vi "synch tester RT.vi"() -> ()   [LabVIEW 2015]
uses:
  <vilib>/rvi/interface/nirviMethod/nirviMethod.xnode
  <vilib>/FPGAPlugInAG/Dynamic/niLvFpga_Run_Dynamic.vi
  <vilib>/FPGAPlugInAG/Dynamic/niLvFpga_ReadFifo_Dynamic.vi
  <vilib>/rvi/errors/niLvFpgaMergeErrorWithErrorCode.vi
  <vilib>/FPGAPlugInAG/Dynamic/niLvFpga_Abort_Dynamic.vi
  <vilib>/rvi/interface/nirviReadWriteControl/nirviReadWriteControl.xnode
  <vilib>/FPGAPlugInAG/Dynamic/niLvFpga_ConfigureFifo_Dynamic.vi
  <vilib>/rvi/interface/nirviOpenFPGA/nirviOpenFPGA.xnode
  <vilib>/FPGAPlugInAG/PXIe-7972R/niLvFpga_Open_PXIe-7972R.vi
  <vilib>/rvi/interface/common/dynamic/niFpgaDynamicAddResources.vi
  NiFpgaLv.dll
  <vilib>/Utility/error.llb/Error Cluster From Error Code.vi
  <vilib>/rvi/interface/Simulation/niFpgaSimulationCallBeginRW.vi
  <vilib>/rvi/errors/niLvFpgaAdjustHostInterfaceError.vi
  FPGA Bitfiles/GMLIDARV5.1_Master_TimingTestermast_BSVpvPZHDb8.lvbitx
  FPGA/Timing Tester master.vi
  FPGA Bitfiles/GMLIDARV5.1_Slave_TimingTesterslav_7ZC0ePWmfic.lvbitx
  FPGA/Timing Tester slave.vi
panel:
  in  "Number of Elements":u32
  out "Elements Remaining":u32
  out "error out 2":errorcluster
  out "error out":errorcluster
  in  "stop":bool
  out "Waveform Graph":i16[](graph)
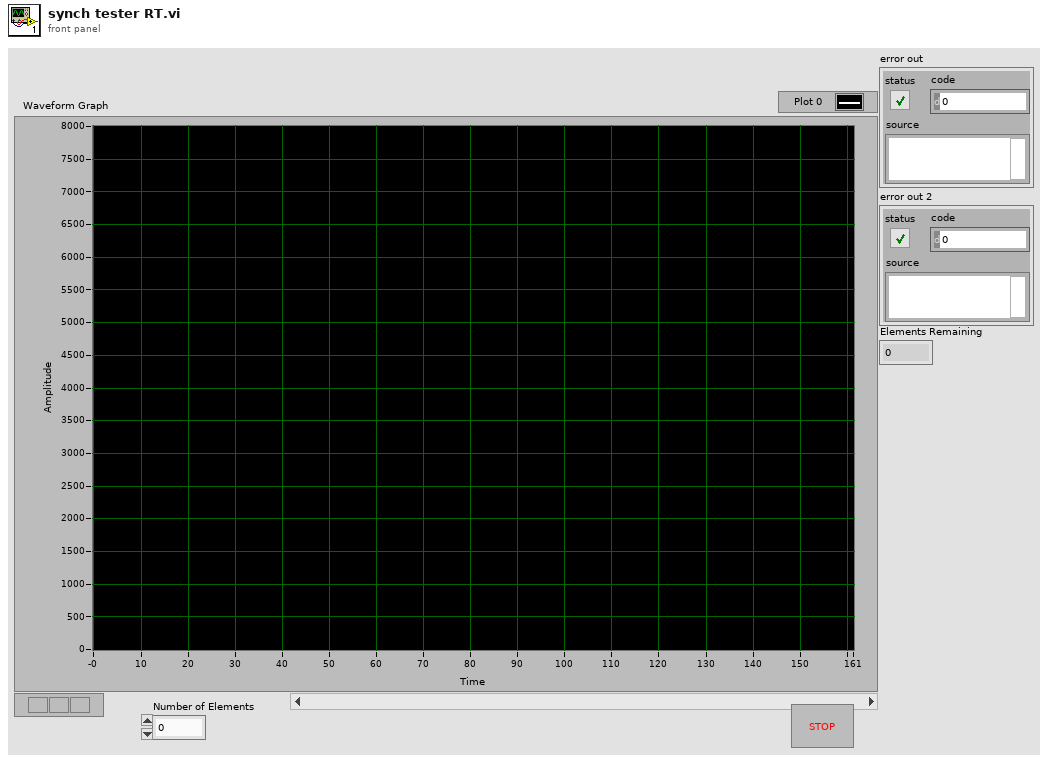
[diagram p1: front panel]
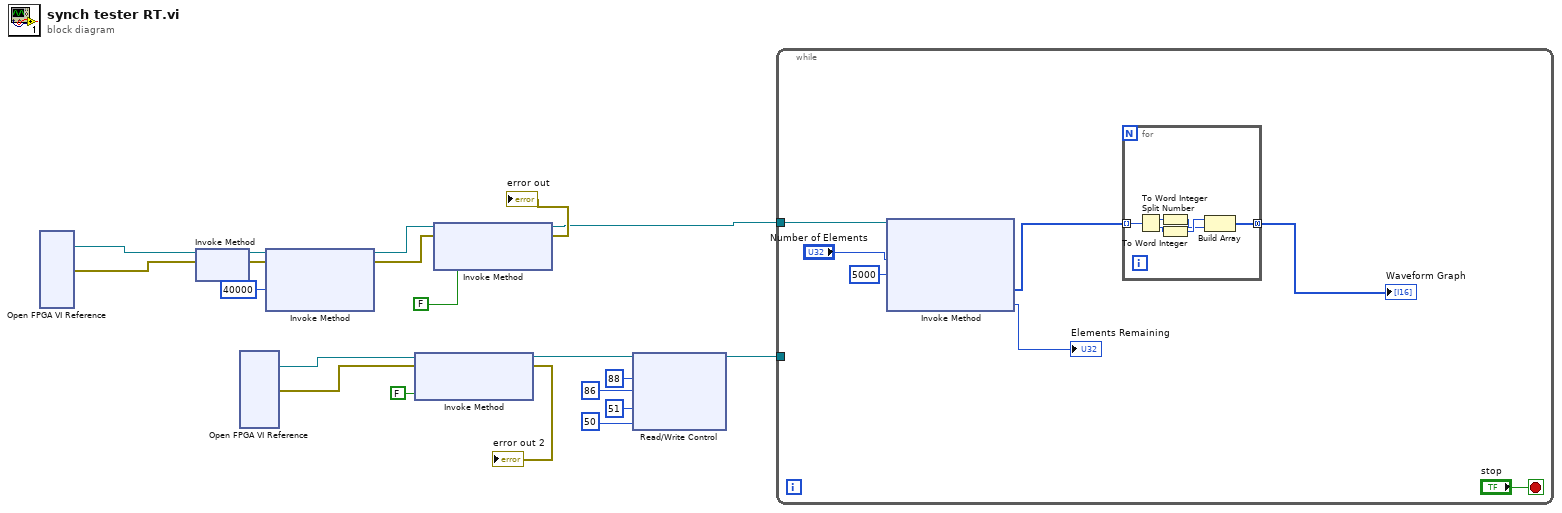
[diagram p0: block diagram]
diagram:
  n1 = xnode "Open FPGA VI Reference"() -> ("FPGA VI Reference Out"=w4:refnum<k20>, "error out"=w1:errorcluster)  [unwired: 2 in]
  n2 = xnode "Invoke Method"("FPGA VI Reference In"=w4, "error in"=w1) -> ("FPGA VI Reference Out"=w16:refnum<k20>, "error out"=w15:errorcluster)
  n3 = xnode "Open FPGA VI Reference"() -> ("FPGA VI Reference Out"=w3:refnum<k20>, "error out"=w2:errorcluster)  [unwired: 2 in]
  n4 = xnode "Invoke Method"("FPGA VI Reference In"=w16, "error in"=w15, "Requested Depth"=u32 40000) -> ("FPGA VI Reference Out"=w13:refnum<k20>, "error out"=w12:errorcluster)  [unwired: 1 out]
  n5 = xnode "Invoke Method"("FPGA VI Reference In"=w3, "error in"=w2, "Wait Until Done (F)"=FALSE) -> ("FPGA VI Reference Out"=w10:refnum<k20>, "error out"=→"error out 2":errorcluster)
  n6 = xnode "Invoke Method"("FPGA VI Reference In"=w13, "error in"=w12, "Wait Until Done (F)"=FALSE) -> ("FPGA VI Reference Out"=w11:refnum<k20>, "error out"=→"error out":errorcluster)
  n7 = xnode "Read/Write Control"("FPGA VI Reference In"=w10, "DOupper limit"=i16 88, "DOlower limit"=i16 86, "AOupper limit"=i16 51, "AOlower limit"=i16 50 ("AOupper limit")) -> ("FPGA VI Reference Out"=w9:refnum<k20>)  [unwired: 1 in, 1 out]
  n8 = while {
    tunnel: w11 -> [w27]
    tunnel: w9 -> [_]
    stop <- "stop" stop-if-true
    n9 = xnode "Invoke Method"("FPGA VI Reference In"=w27, "Number of Elements"="Number of Elements", "Timeout (ms)"=5000) -> ("Data"=w22:u32[], "Elements Remaining"=→"Elements Remaining":u32)  [unwired: 1 in, 2 out]
    n10 = for {
      tunnel: w22 -> [w31] mode=indexing
      tunnel: [w30] -> w21 mode=concatenating
      n11 = Split Number(x=w31) -> (hi(x)=w33:u16, lo(x)=w32:u16)
      n12 = To Word Integer(number=w33) -> (16bit integer=w28:i16)
      n13 = To Word Integer(number=w32) -> (16bit integer=w29:i16)
      n14 = Build Array(w29, w28) -> (w30:i16[])
    }
    "Waveform Graph" <- w21
  }
